vi "Loop.vi"() -> ()   [LabVIEW 2017, in "tmp.lvlib"]
uses:
  tmp.lvlib
  Communication/MsgError.ctl
  Communication/Communication.lvlib
panel:
  out "data":T1
  out "current time":timestamp
  out "Data":variant
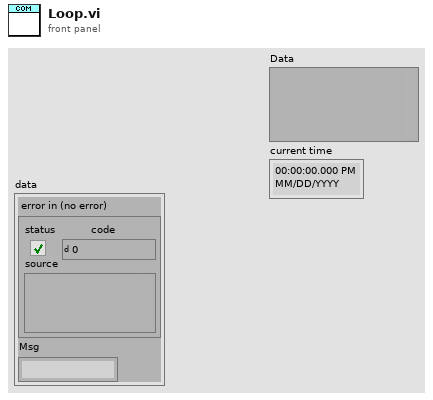
[diagram p1: front panel]
types:
  T1 = typedef "Communication.lvlib/MsgError.ctl" = cluster{"error in (no error)":errorcluster, "Msg":string}
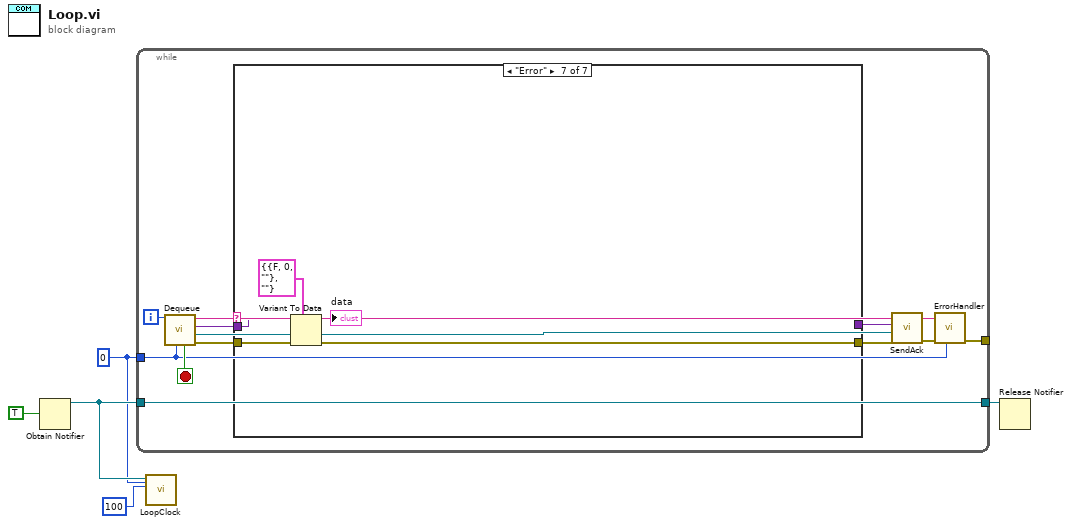
[diagram p0: block diagram]
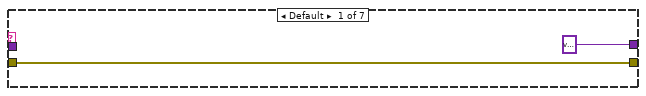
[diagram p2: hidden frame]
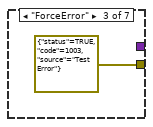
[diagram p4: hidden frame]
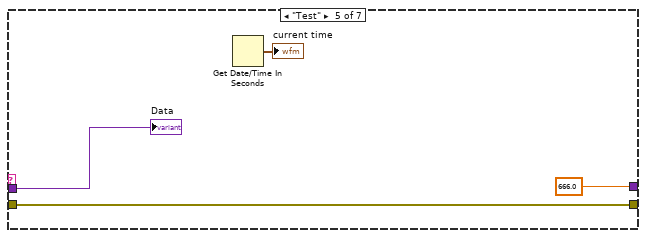
[diagram p6: hidden frame]
diagram:
  w1 = 0
  n1 = Obtain Notifier(notification data type=TRUE) -> (notifier out=w5:refnum<notifier>)  [unwired: 3 in, 2 out]
  n2 = while {
    tunnel: w5 -> [w15]
    tunnel: [w15] -> w3
    tunnel: w1 -> [w8]
    tunnel: [w10] -> _
    i -> [w9]
    stop <- w17 stop-if-true
    n3 = call "Dequeue.vi"("Instance"=w8, "Loop Counter"=w9) -> ("error out"=w13:errorcluster, "ResponseNotifcation"=w14:refnum<notifier>, "Data"=w16:variant, "Msg"=w7:string, "Exit?"=w17:bool)  [unwired: 5 in]
    n4 = case shown="\"Error\"" w7 {
      tunnel: w16 -> [_ _ _ _ w26 _ w31]
      tunnel: w13 -> [w19 w20 _ w22 w24 w27 w32]
      tunnel: [variant _ _ _ 666.0 _ _] -> w12
      tunnel: [w19 w20 errorcluster {"status"=TRUE, "code"=1003, "source"="Test Error"} ("error in (no error)") w22 w24 w27 w28] -> w6
      frame Default {
      }
      frame "Init" {
      }
      frame "ForceError" {
      }
      frame "Exit" {
      }
      frame "Test" {
        n5 = Get Date/Time In Seconds() -> (seconds since 1Jan1904=→"current time":timestamp)
        "Data" <- w26
      }
      frame "Tick" {
      }
      frame "Error" {
        n6 = Variant To Data(error in=w32, type=T1 {"error in (no error)"={"status"=FALSE, "code"=0, "source"=""}, "Msg"=""} ("Cluster"), Variant=w31) -> (data=→"data":T1, error out=w28:errorcluster)
      }
    }
    n7 = call "SendAck.vi"("error in (no error)"=w6, "Ack"=w14, "Variant"=w12) -> ("error out"=w11:errorcluster)  [unwired: 8 in]
    n8 = call "ErrorHandler.vi"("Instance"=w8, "error in (no error)"=w11, "Msg"=w7) -> ("error out"=w10:errorcluster)  [unwired: 8 in]
  }
  n9 = call "LoopClock.vi"("Instance"=w1, "timeout in ms (-1)"=100, "Notifier in"=w5) -> ()  [unwired: 9 in]
  n10 = Release Notifier(notifier=w3) -> ()  [unwired: 2 in, 3 out]
